vi "Read Igor Commands.vi"(8 "error in (no error)":errorcluster, 11 "Data Save":refnum<class "Data.lvclass">) -> (0 "error out":errorcluster, 2 "Igor Commands":string, 3 "Data Save out":refnum<class "Data.lvclass">)   [LabVIEW 2019, in "Data.lvclass"]
uses:
  Data.lvclass
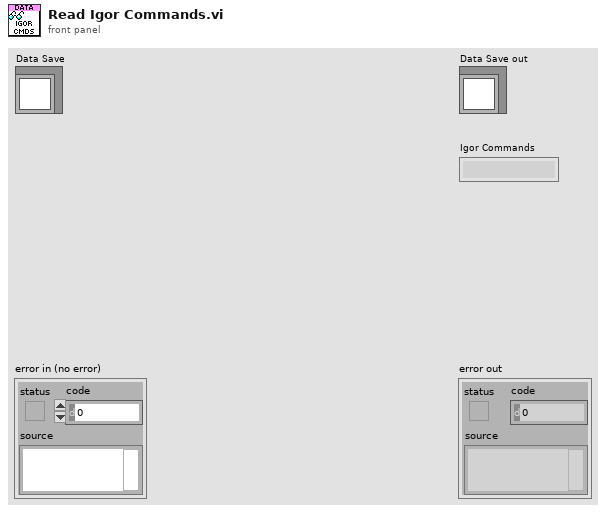
[diagram p1: front panel]
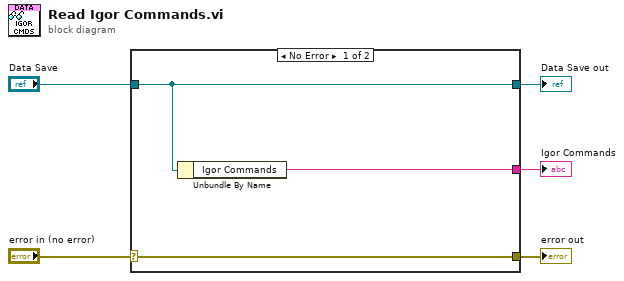
[diagram p0: block diagram]
diagram:
  n1 = case shown="No Error" "error in (no error)" {
    selector: "error in (no error)" -> [w8 w9]
    tunnel: [w8 w9] -> w4
    tunnel: [w7 w10] -> w2
    tunnel: "Data Save" -> [w7 w10]
    tunnel: [w6 _] -> w1
    frame No Error {
      n2 = Unbundle By Name(w7) -> ("Igor Commands"=w6:string)
    }
    frame Error {
    }
  }
  "error out" <- w4
  "Data Save out" <- w2
  "Igor Commands" <- w1
